vi "After Reset Delay.vi"(6 "Startup delay (0 ms)":u32, 7 "Skip delay? (F)":bool, 8 "error in":errorcluster) -> (0 "error out":errorcluster)   [LabVIEW 2020, in "QuPMXdriver.lvlib"]
doc: "Delay required after start up or reset of the device.\nIn case of error the delay is always skipped.\nAfter initalization of communication (even before sending command, simple VISA open is sufficient), some microcontrolers resets itself because of DTR signal is tied to reset in a bad way. Because of this an additional time is needed before sending first command, to wait till reset finish."
uses:
  QuPMXdriver.lvlib
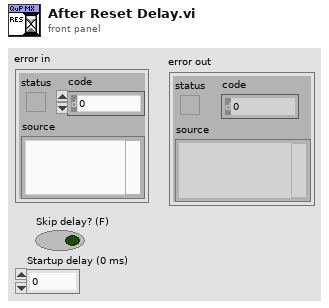
[diagram p1: front panel]
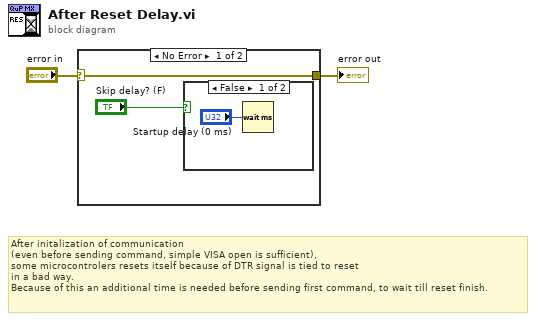
[diagram p0: block diagram]
diagram:
  # "After initalization of communication\n(even before sending command, simple VISA open is sufficient),\nsome microcontrolers resets itself because of DTR signal is tied to reset\nin a bad way.\nBecause of this an additional time is needed before sending first command, to wait till reset finish."
  n1 = case shown="No Error" "error in" {
    selector: "error in" -> [w3 w6]
    tunnel: [w3 w6] -> w1
    frame No Error {
      n2 = case shown="False" "Skip delay? (F)" {
        frame False {
          n3 = Wait (ms)(milliseconds to wait="Startup delay (0 ms)") -> ()  [unwired: 1 out]
        }
        frame True {
        }
      }
    }
    frame Error {
    }
  }
  "error out" <- w1
